vi "Actor Core.vi"(8 "error in":errorcluster, 11 "Hardware in":refnum<class "galvo_panel.lvclass">) -> (0 "error out":errorcluster, 3 "Actor out":refnum<class "Actor.lvclass">)   [LabVIEW 2015, in "galvo_panel.lvclass"]
doc: "(<B>Filename</B>: Actor Framework.lvlib:Actor.lvclass:Actor Core.vi)\n\nReceives messages to the actor, reacts to them, and initiates any error handling that may shut the actor down.\n\nDescendant classes may override this VI to append parallel tasks for the actor to complete while it handles messages. Overrides use the Call Parent Method node."
uses:
  galvo_panel.lvclass
  <vilib>/ActorFramework/Actor/Actor.lvclass
  UI/panel_class/panel.lvclass/panel.ctl
  <vilib>/ActorFramework/Actor/Actor.lvclass/Actor.ctl
  <vilib>/ActorFramework/Message Enqueuer/Message Enqueuer.lvclass/Message Enqueuer.ctl
  galvo_panel Messages/gpanel_move_xy Msg/gpanel_move_xy Msg.lvclass/gpanel_move_xy Msg.ctl
  galvo_panel Messages/gpanel_set_physical_chennels_xy Msg/gpanel_set_physical_chennels_xy Msg.lvclass/gpanel_set_physical_chennels_xy Msg.ctl
  <vilib>/ActorFramework/Message Enqueuer/Init from Existing Queue.vi
  <vilib>/ActorFramework/Message Enqueuer/Enqueue.vi
  <vilib>/ActorFramework/Message Priority Queue/Priority Enqueue.vi
  cursor_global.vi
  <vilib>/ActorFramework/Message Enqueuer/Message Enqueuer.lvclass
  galvo_panel Messages/gpanel_move_xy Msg/gpanel_move_xy Msg.lvclass
  galvo_panel Messages/gpanel_set_physical_chennels_xy Msg/gpanel_set_physical_chennels_xy Msg.lvclass
  UI/panel_class/panel.lvclass
  <vilib>/Utility/file.llb/Read Delimited Spreadsheet (DBL).vi
panel:
  in  "stop":bool
  in  "Listbox":i32(listbox)
  in  "movee":bool
  in  "Track Cursor":bool
  in  "inc":dbl
  in  "left":bool
  in  "right":bool
  in  "down":bool
  in  "up":bool
  in  "copy_map_coors":bool
  out "Status":string
  in  "Move":bool
  in  "Y Position":dbl min=-10.0 max=10.0
  in  "X Position":dbl min=-10.0 max=10.0
  in  "X Channel":tag
  in  "Y Channel":tag
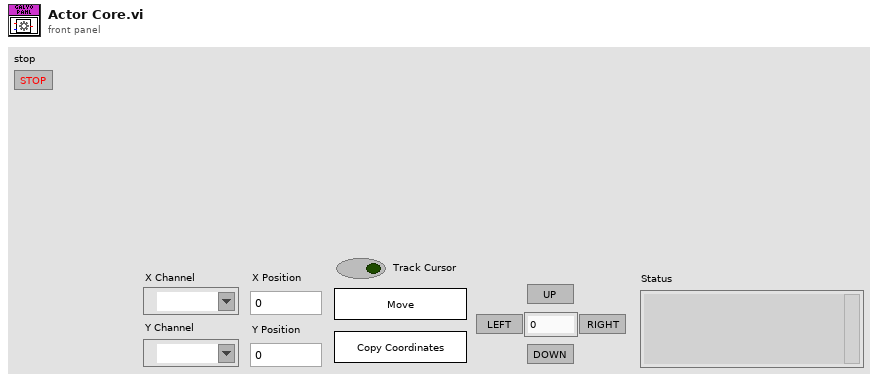
[diagram p1: front panel]
types:
  T1 = typedef "galvo_event_refs.ctl" = cluster{"update_galvo_status":refnum<event-registration>}
  T2 = cluster{"update_galvo_status":refnum<event-registration>, "stop_ui_ref":refnum<event-registration>}
  T3 = typedef "ui_plot_references.ctl" = cluster{"plots":refnum<vi>, "chart":refnum<vi>, "graph":refnum<vi>, "map":refnum<vi>, "XY Graph":refnum<vi>}
  T4 = typedef "LVPointDoubleTypeDef.ctl" = cluster{"Cursor X":dbl, "Cursor Y":dbl}
  T5 = typedef "ui_elements.ctl" = cluster{"map_xcursor":refnum<vi>, "map_ycursor":refnum<vi>}
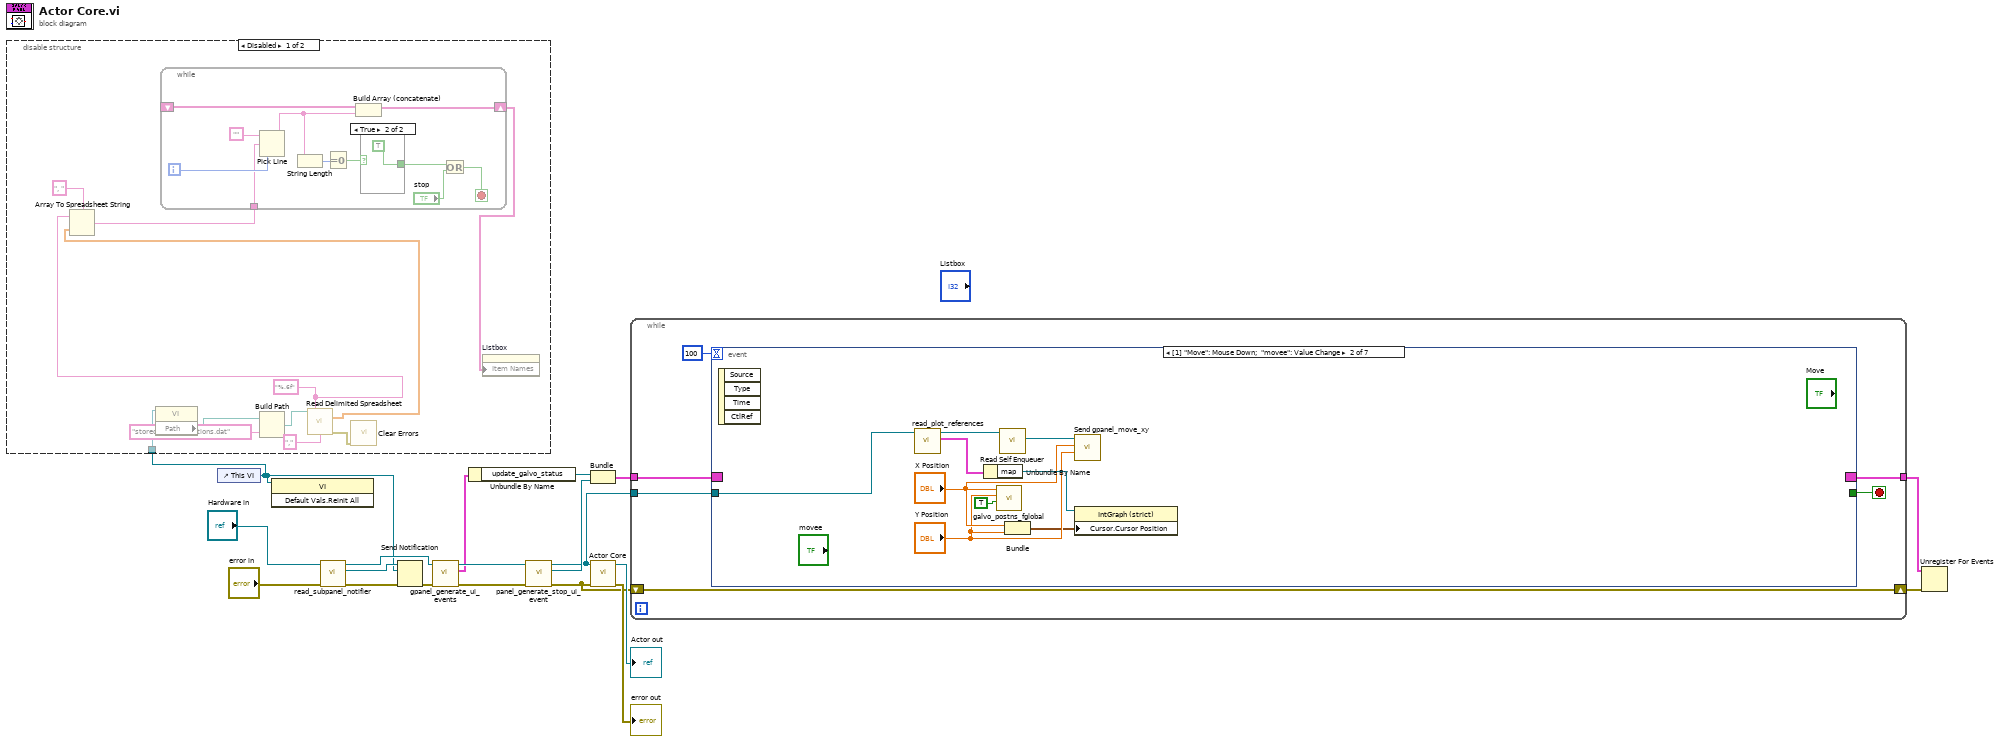
[diagram p0: block diagram]
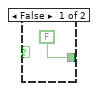
[diagram p2: hidden frame]
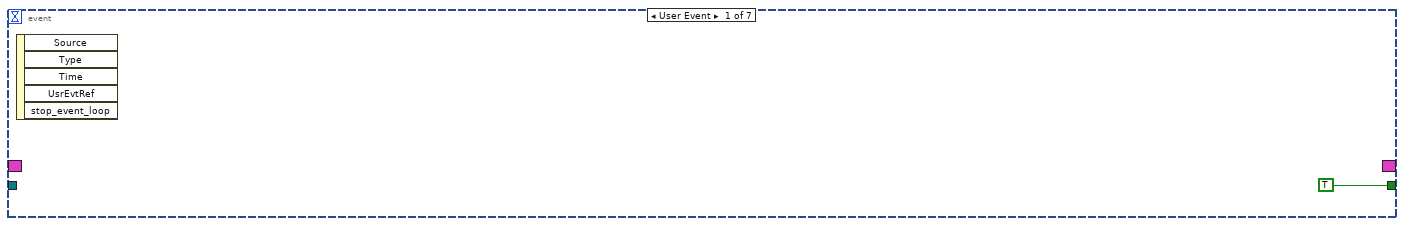
[diagram p4: hidden frame]
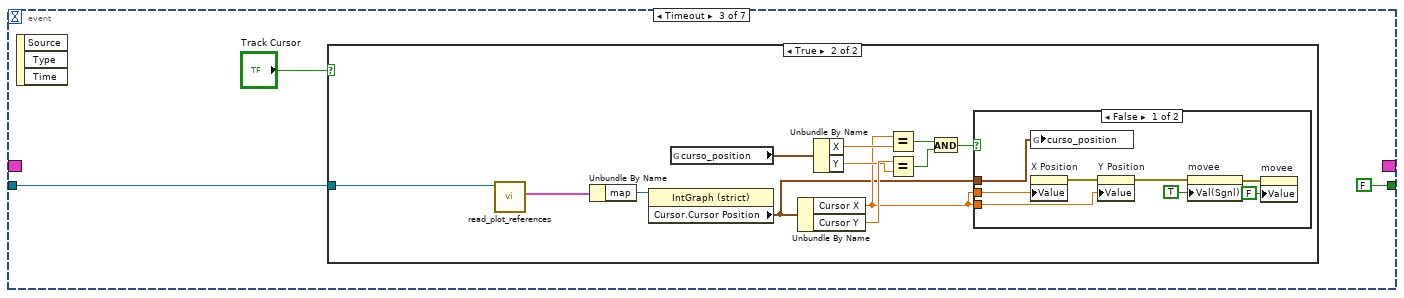
[diagram p5: hidden frame]
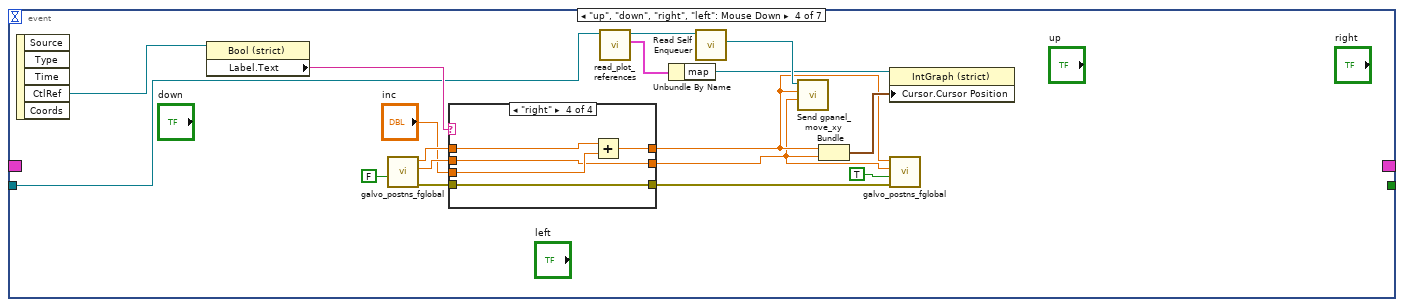
[diagram p8: hidden frame]
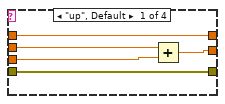
[diagram p9: hidden frame]
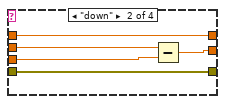
[diagram p10: hidden frame]
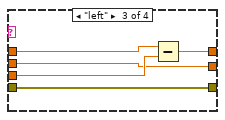
[diagram p11: hidden frame]
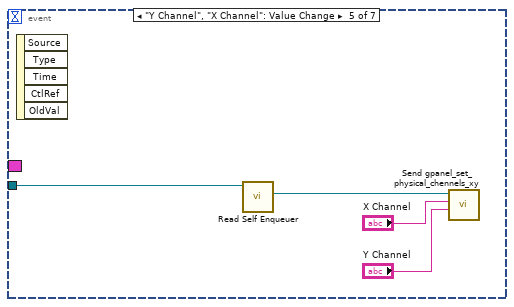
[diagram p12: hidden frame]
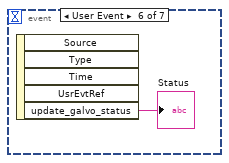
[diagram p13: hidden frame]
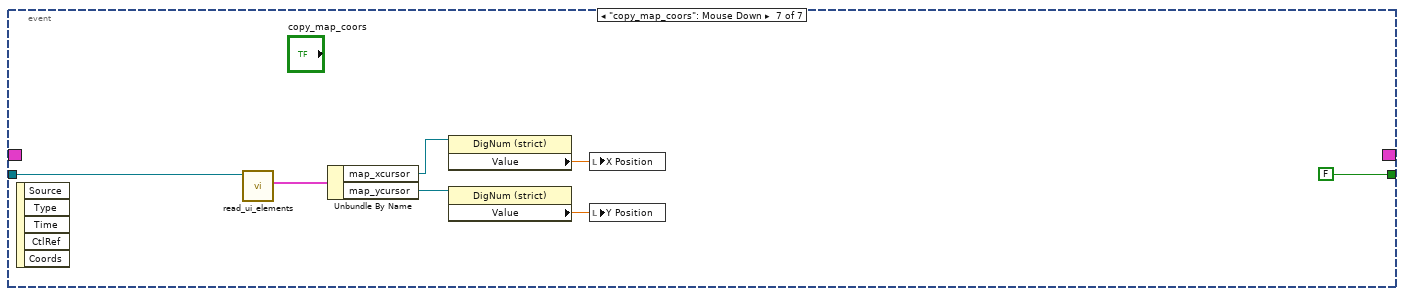
[diagram p14: hidden frame]
diagram:
  n1 = control-ref of="This VI"() -> (w1:refnum<vi>)
  n2 = disable-structure shown="Disabled" {
    disable-tunnel: w1 -> [w30 _]
    frame Disabled {
      w21 = "%.6f" ("format (%.3f)")
      n3 = property class="VI"(reference=w30) -> ("Path"=w29:path)  [unwired: 1 in, 2 out]
      n4 = Build Path(base path=w29, name or relative path="stored_galvo_positions.dat") -> (appended path=w27:path)
      n5 = call-poly <vilib>:"Read Delimited Spreadsheet.vi"("file path (dialog if empty)"=w27, "format (%.3f)"=w21, "delimiter (\\t)"="," ("delimiter (\\t)")) -> ("all rows"=w22:dbl[][], "error out"=w26:errorcluster)  [unwired: 7 in, 4 out]
      n6 = Array To Spreadsheet String(delimiter (Tab)=", ", array=w22, 3:w21) -> (spreadsheet string=w24:string)
      n7 = while {
        shift-right: [w39] -> w20
        shift-left: _ -> [w40]
        tunnel: w24 -> [w31]
        i -> [w41]
        stop <- w32 stop-if-true
        n8 = Pick Line(string ("")="", multi-line string=w31, line index=w41) -> (output string=w37:string)
        n9 = String Length(string=w37) -> (length=w36:i32)
        n10 = Equal To 0?(x=w36) -> (x = 0?=w35:bool)
        n11 = Build Array (concatenate)(w40, w37) -> (w39:string[])
        n12 = case shown="True" w35 {
          tunnel: [FALSE TRUE] -> w34
          frame False {
          }
          frame True {
          }
        }
        n13 = Or(x=w34, y="stop") -> (x .or. y?=w32:bool)
      }
      n14 = call <vilib>:"Clear Errors.vi"("error in (no error)"=w26) -> ()  [unwired: 5 in, 2 out]
      n15 = property on="Listbox" class="LstBox (strict)"("Item Names"=w20) -> ()  [unwired: 2 in, 2 out]
    }
    frame Enabled {
    }
  }
  n16 = invoke class="VI" method="Default Vals.Reinit All"(reference=w1) -> ()  [unwired: 2 in, 3 out]
  n17 = call "read_subpanel_notifier.vi"("error in (no error)"="error in", "panel in"="Hardware in") -> ("error out"=w15:errorcluster, "subpanel_notifier"=w16:refnum<notifier>, "panel out"=w9:refnum<class "galvo_panel.lvclass">)  [unwired: 7 in]
  n18 = Send Notification(notification=w1, notifier=w16, error in (no error)=w15) -> (error out=w11:errorcluster)  [unwired: 1 out]
  n19 = call "gpanel_generate_ui_events.vi"("error in (no error)"=w11, "galvo_panel in"=w9) -> ("error out"=w10:errorcluster, "ui_events"=w7:T1, "galvo_panel out"=w8:refnum<class "galvo_panel.lvclass">)  [unwired: 7 in]
  n20 = Unbundle By Name(w7) -> ("update_galvo_status"=w6:refnum<event-registration>)
  n21 = call "panel_generate_stop_ui_event.vi"("error in (no error)"=w10, "panel in"=w8) -> ("error out"=w12:errorcluster, "stop_ui_ref"=w5:refnum<event-registration>, "panel out"=w2:refnum<class "galvo_panel.lvclass">)  [unwired: 7 in]
  n22 = Bundle("update_galvo_status"=w6, "stop_ui_ref"=w5) -> (w4:T2)  [unwired: 1 in]
  n23 = call-parent "Actor Core.vi"("error in"=w12, "Actor in"=w2) -> ("error out"=→"error out":errorcluster, "Actor out"=→"Actor out":refnum<class "Actor.lvclass">)  [unwired: 8 in]
  n24 = while {
    tunnel: w4 -> [w49]
    tunnel: [w47] -> w13
    shift-right: [w46] -> w3
    shift-left: w12 -> [w46]
    tunnel: w2 -> [w45]
    stop <- w48 stop-if-true
    n25 = event shown="[1] \"Move\": Mouse Down;  \"movee\": Value Change" {
      selector: w49 -> [_ _ _ _ _ _ _]
      dyn-events: [_ _ _ _ _ _ _] -> w47
      timeout: 100 -> [_ _ _ _ _ _ _]
      tunnel: [TRUE _ FALSE _ _ _ FALSE] -> w48
      tunnel: w45 -> [_ w55 w61 w89 w123 _ w131]
      event User Event {
        n26 = event-data() -> ()  [unwired: 1 in, 5 out]
      }
      event "Move": Mouse Down; "movee": Value Change {
        n27 = event-data() -> ()  [unwired: 1 in, 4 out]
        n28 = call "read_plot_references.vi"("panel in"=w55) -> ("plot_references"=w57:T3, "panel out"=w54:refnum<class "galvo_panel.lvclass">)  [unwired: 8 in, 1 out]
        n29 = Unbundle By Name(w57) -> ("map"=w56:refnum<vi>)
        n30 = call "galvo_postns_fglobal.vi"("write?"=TRUE, "curr_y"="Y Position", "curr_x"="X Position") -> ()  [unwired: 6 in, 3 out]
        n31 = call <vilib>:"Read Self Enqueuer.vi"("Actor"=w54) -> ("Self Enqueuer"=w59:refnum<class "Message Enqueuer.lvclass">)  [unwired: 10 in]
        n32 = Bundle("X Position"="X Position", "Y Position"="Y Position") -> (w51:cluster{"X Position":dbl, "Y Position":dbl})  [unwired: 1 in]
        n33 = call "Send gpanel_move_xy.vi"("Y Position"="Y Position", "X Position"="X Position", "Message Enqueuer"=w59) -> ()  [unwired: 7 in, 2 out]
        n34 = property class="IntGraph (strict)"(reference=w56, "Cursor.Cursor Position"=w51) -> ()  [unwired: 1 in, 2 out]
      }
      event Timeout {
        n35 = event-data() -> ()  [unwired: 1 in, 3 out]
        n36 = case shown="True" "Track Cursor" {
          tunnel: w61 -> [_ w73]
          frame False {
          }
          frame True {
            n37 = call "read_plot_references.vi"("panel in"=w73) -> ("plot_references"=w74:T3)  [unwired: 8 in, 2 out]
            n38 = Unbundle By Name(w74) -> ("map"=w72:refnum<vi>)
            n39 = property class="IntGraph (strict)"(reference=w72) -> ("Cursor.Cursor Position"=w63:T4)  [unwired: 1 in, 2 out]
            n40 = global read "cursor_global.vi" "curso_position"() -> (w71:T4)
            n41 = Unbundle By Name(w63) -> ("Cursor X"=w64:dbl, "Cursor Y"=w69:dbl)
            n42 = Unbundle By Name(w71) -> ("X"=w70:dbl, "Y"=w68:dbl)
            n43 = Equal?(x=w64, y=w70) -> (x = y?=w66:bool)
            n44 = Equal?(x=w69, y=w68) -> (x = y?=w67:bool)
            n45 = And(x=w66, y=w67) -> (x .and. y?=w65:bool)
            n46 = case shown="False" w65 {
              tunnel: w64 -> [w82 _]
              tunnel: w64 -> [w81 _]
              tunnel: w63 -> [w79 _]
              frame False {
                n47 = global write "cursor_global.vi" "curso_position"(w79) -> ()
                n48 = property on="X Position" class="DigNum (strict)"("Value"=w82) -> (error out=w80:errorcluster)  [unwired: 2 in, 1 out]
                n49 = property on="Y Position" class="DigNum (strict)"(error in=w80, "Value"=w81) -> (error out=w78:errorcluster)  [unwired: 1 in, 1 out]
                n50 = property on="movee" class="Bool (strict)"(error in=w78, "Val(Sgnl)"=TRUE ("Value (Signaling)")) -> (error out=w76:errorcluster)  [unwired: 1 in, 1 out]
                n51 = property on="movee" class="Bool (strict)"(error in=w76, "Value"=FALSE ("movee")) -> ()  [unwired: 1 in, 2 out]
              }
              frame True {
              }
            }
          }
        }
      }
      event "up", "down", "right", "left": Mouse Down {
        n52 = event-data() -> ("CtlRef"=w97:refnum<vi>)  [unwired: 1 in, 4 out]
        n53 = property class="Bool (strict)"(reference=w97) -> ("Label.Text"=w96:string)  [unwired: 1 in, 2 out]
        n54 = call "galvo_postns_fglobal.vi"("write?"=FALSE) -> ("error out"=w91:errorcluster, "curr_y"=w94:dbl, "curr_x"=w95:dbl)  [unwired: 8 in]
        n55 = case shown="\"right\"" w96 {
          tunnel: w95 -> [w102 w106 w114 w119]
          tunnel: w94 -> [w103 w108 w111 w116]
          tunnel: "inc" -> [w104 w109 w113 w118]
          tunnel: [w102 w106 w112 w117] -> w84
          tunnel: [w101 w107 w111 w116] -> w83
          tunnel: w91 -> [w100 w105 w110 w115]
          tunnel: [w100 w105 w110 w115] -> w90
          frame "up", Default {
            n56 = Add(x=w103, y=w104) -> (x+y=w101:dbl)
          }
          frame "down" {
            n57 = Subtract(x=w108, y=w109) -> (x-y=w107:dbl)
          }
          frame "left" {
            n58 = Subtract(x=w114, y=w113) -> (x-y=w112:dbl)
          }
          frame "right" {
            n59 = Add(x=w119, y=w118) -> (x+y=w117:dbl)
          }
        }
        n60 = call "read_plot_references.vi"("panel in"=w89) -> ("plot_references"=w87:T3, "panel out"=w88:refnum<class "galvo_panel.lvclass">)  [unwired: 8 in, 1 out]
        n61 = Unbundle By Name(w87) -> ("map"=w86:refnum<vi>)
        n62 = call <vilib>:"Read Self Enqueuer.vi"("Actor"=w88) -> ("Self Enqueuer"=w99:refnum<class "Message Enqueuer.lvclass">)  [unwired: 10 in]
        n63 = call "Send gpanel_move_xy.vi"("Y Position"=w83, "X Position"=w84, "Message Enqueuer"=w99) -> ()  [unwired: 7 in, 2 out]
        n64 = Bundle("curr_x"=w84, "curr_y"=w83) -> (w85:cluster{"curr_x":dbl, "curr_y":dbl})  [unwired: 1 in]
        n65 = property class="IntGraph (strict)"(reference=w86, "Cursor.Cursor Position"=w85) -> ()  [unwired: 1 in, 2 out]
        n66 = call "galvo_postns_fglobal.vi"("error in (no error)"=w90, "write?"=TRUE, "curr_y"=w83, "curr_x"=w84) -> ()  [unwired: 5 in, 3 out]
      }
      event "Y Channel", "X Channel": Value Change {
        n67 = event-data() -> ()  [unwired: 1 in, 5 out]
        n68 = call <vilib>:"Read Self Enqueuer.vi"("Actor"=w123) -> ("Self Enqueuer"=w122:refnum<class "Message Enqueuer.lvclass">)  [unwired: 10 in]
        n69 = call "Send gpanel_set_physical_chennels_xy.vi"("Y Channel"="Y Channel", "X Channel"="X Channel", "Message Enqueuer"=w122) -> ()  [unwired: 7 in, 2 out]
      }
      event User Event {
        n70 = event-data() -> ("update_galvo_status"=→"Status":string)  [unwired: 1 in, 4 out]
      }
      event "copy_map_coors": Mouse Down {
        n71 = event-data() -> ()  [unwired: 1 in, 5 out]
        n72 = call "read_ui_elements.vi"("panel in"=w131) -> ("ui_elements"=w130:T5)  [unwired: 8 in, 2 out]
        n73 = Unbundle By Name(w130) -> ("map_xcursor"=w129:refnum<vi>, "map_ycursor"=w127:refnum<vi>)
        n74 = property class="DigNum (strict)"(reference=w129) -> ("Value"=w128:dbl)  [unwired: 1 in, 2 out]
        n75 = property class="DigNum (strict)"(reference=w127) -> ("Value"=w126:dbl)  [unwired: 1 in, 2 out]
        n76 = local write "X Position"(w128) -> ()
        n77 = local write "Y Position"(w126) -> ()
      }
    }
  }
  n78 = Unregister For Events(event registration refnum=w13, error in=w3) -> ()  [unwired: 1 out]
